vi "piezoWriteClose.vi"   [LabVIEW 2017]
uses:
  <vilib>/DAQmx/read.llb/DAQmx Read (Analog DBL 1Chan 1Samp).vi
  <vilib>/DAQmx/write.llb/DAQmx Write (Analog DBL 1Chan 1Samp).vi
  globalDevices.vi
  <vilib>/DAQmx/create/channels.llb/DAQmx Create Channel (AI-Voltage-Basic).vi
  <vilib>/DAQmx/miscellaneous.llb/DAQmx Fill In Error Info.vi
  <vilib>/DAQmx/create/channels.llb/DAQmx Create Channel (AO-Voltage-Basic).vi
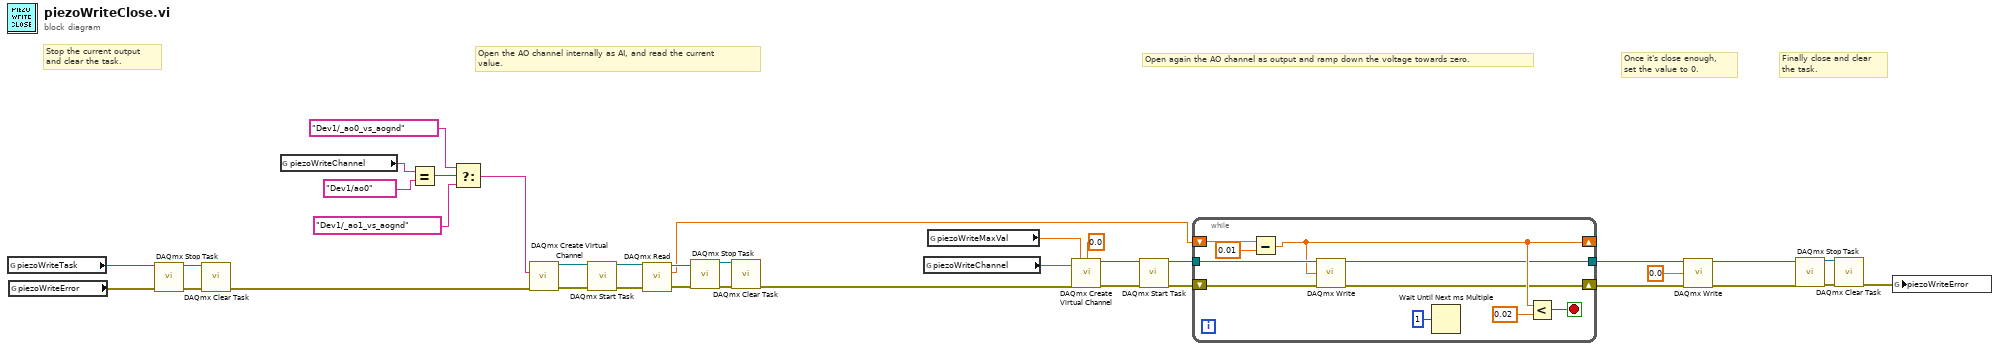
[diagram p0: block diagram]
diagram:
  # "Finally close and clear\nthe task."
  # "Once it's close enough,\nset the value to 0."
  # "Open again the AO channel as output and ramp down the voltage towards zero."
  # "Open the AO channel internally as AI, and read the current\nvalue."
  # "Stop the current output\nand clear the task."
  n1 = global read "globalDevices.vi" "piezoWriteTask"() -> (w35:refnum<k21>)
  n2 = global read "globalDevices.vi" "piezoWriteError"() -> (w36:errorcluster)
  n3 = call <vilib>:"DAQmx Stop Task.vi"("task/channels in"=w35, "error in"=w36) -> ("task out"=w33:refnum<k21>, "error out"=w34:errorcluster)  [unwired: 12 in]
  n4 = call <vilib>:"DAQmx Clear Task.vi"("task in"=w33, "error in"=w34) -> ("error out"=w12:errorcluster)  [unwired: 13 in]
  n5 = global read "globalDevices.vi" "piezoWriteChannel"() -> (w18:tag)
  n6 = Equal?(x=w18, y=tag "Dev1/ao0" ("physical channels")) -> (x = y?=w16:bool)
  n7 = Select(t=tag "Dev1/_ao0_vs_aognd" ("physical channels"), s=w16, f=tag "Dev1/_ao1_vs_aognd" ("physical channels")) -> (s? t:f=w13:tag)
  n8 = call-poly <vilib>:"DAQmx Create Virtual Channel.vi"("physical channels"=w13, "error in"=w12) -> ("task out"=w24:refnum<k21>, "error out"=w11:errorcluster)  [unwired: 12 in]
  n9 = call <vilib>:"DAQmx Start Task.vi"("task/channels in"=w24, "error in"=w11) -> ("task out"=w23:refnum<k21>, "error out"=w10:errorcluster)  [unwired: 12 in]
  n10 = call-poly <vilib>:"DAQmx Read.vi"("task/channels in"=w23, "error in"=w10) -> ("task out"=w22:refnum<k21>, "data"=w20:dbl, "error out"=w9:errorcluster)  [unwired: 11 in]
  n11 = call <vilib>:"DAQmx Stop Task.vi"("task/channels in"=w22, "error in"=w9) -> ("task out"=w26:refnum<k21>, "error out"=w25:errorcluster)  [unwired: 12 in]
  n12 = call <vilib>:"DAQmx Clear Task.vi"("task in"=w26, "error in"=w25) -> ("error out"=w21:errorcluster)  [unwired: 13 in]
  n13 = global read "globalDevices.vi" "piezoWriteChannel"() -> (w19:tag)
  n14 = global read "globalDevices.vi" "piezoWriteMaxVal"() -> (w27:dbl)
  n15 = call-poly <vilib>:"DAQmx Create Virtual Channel.vi"("maximum value"=w27, "minimum value"=0.0, "physical channels"=w19, "error in"=w21) -> ("task out"=w29:refnum<k21>, "error out"=w8:errorcluster)  [unwired: 10 in]
  n16 = call <vilib>:"DAQmx Start Task.vi"("task/channels in"=w29, "error in"=w8) -> ("task out"=w28:refnum<k21>, "error out"=w7:errorcluster)  [unwired: 12 in]
  n17 = while {
    shift-right: [w41] -> _
    shift-left: w20 -> [w46]
    tunnel: w28 -> [w42]
    tunnel: [w40] -> w6
    shift-right: [w37] -> w5
    shift-left: w7 -> [w38]
    stop <- w43 stop-if-true
    n18 = Subtract(x=w46, y=0.01) -> (x-y=w41:dbl)
    n19 = call-poly <vilib>:"DAQmx Write.vi"("task/channels in"=w42, "data"=w41, "error in"=w38) -> ("task out"=w40:refnum<k21>, "error out"=w37:errorcluster)  [unwired: 10 in, 1 out]
    n20 = Wait Until Next ms Multiple(millisecond multiple=u32 1) -> ()  [unwired: 1 out]
    n21 = Less?(x=w41, y=0.02) -> (x < y?=w43:bool)
  }
  n22 = call-poly <vilib>:"DAQmx Write.vi"("task/channels in"=w6, "data"=0.0, "error in"=w5) -> ("task out"=w4:refnum<k21>, "error out"=w3:errorcluster)  [unwired: 10 in, 1 out]
  n23 = call <vilib>:"DAQmx Stop Task.vi"("task/channels in"=w4, "error in"=w3) -> ("task out"=w32:refnum<k21>, "error out"=w31:errorcluster)  [unwired: 12 in]
  n24 = call <vilib>:"DAQmx Clear Task.vi"("task in"=w32, "error in"=w31) -> ("error out"=w1:errorcluster)  [unwired: 13 in]
  n25 = global write "globalDevices.vi" "piezoWriteError"(w1) -> ()
